vi "Set Loop Period.vi"(8 "error in (no error)":errorcluster, 10 "loop period":u32, 11 "PID Controller in":refnum<class "PID Controller.lvclass">) -> (0 "error out":errorcluster, 3 "PID Controller out":refnum<class "PID Controller.lvclass">)   [LabVIEW 2024, in "PID Controller.lvlib" / "PID Controller.lvclass"]
uses:
  PID Controller.lvclass
  PID Controller.lvclass/PID Controller.ctl
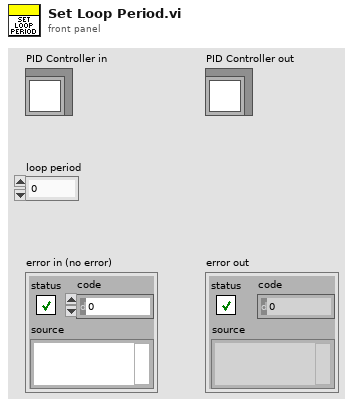
[diagram p1: front panel]
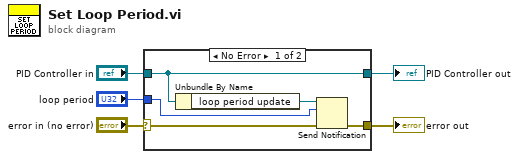
[diagram p0: block diagram]
diagram:
  n1 = case shown="No Error" "error in (no error)" {
    selector: "error in (no error)" -> [w7 w12]
    tunnel: [w6 w12] -> w4
    tunnel: [w8 w11] -> w2
    tunnel: "PID Controller in" -> [w8 w11]
    tunnel: "loop period" -> [w10 _]
    frame No Error {
      n2 = Unbundle By Name(w8) -> ("loop period update"=w9:refnum<notifier>)
      n3 = Send Notification(notification=w10, notifier=w9, error in (no error)=w7) -> (error out=w6:errorcluster)  [unwired: 1 out]
    }
    frame Error {
    }
  }
  "error out" <- w4
  "PID Controller out" <- w2
